vi "GEA2 Send Message.vi"(0 "GEA2 Reference In":refnum<k24>, 1 "Input Data":T1 {"Command" format="%02x"; "Destination" format="%02x"; "Source" format="%02x"}, 2 "Retry Count":u32=3, 11 "Error In":errorcluster) -> (4 "GEA2 Reference Out":refnum<k24>, 15 "Error Out":errorcluster)   [LabVIEW 2016, in "GEA2_Toolkit.lvlib"]
doc: "This VI sends a GEA2 message accross the GEA2 bus."
uses:
  library/GEA2_Toolkit.lvlib
  type defs/Data In.ctl
  C:/Technology Lab/NI-2010/Trunk/Utility/LabVIEW GEA2 Toolkit v1.0.0.0/Appliance.NET/GeaCommunication.dll
  Appliance.NET/GeaCommunication.dll
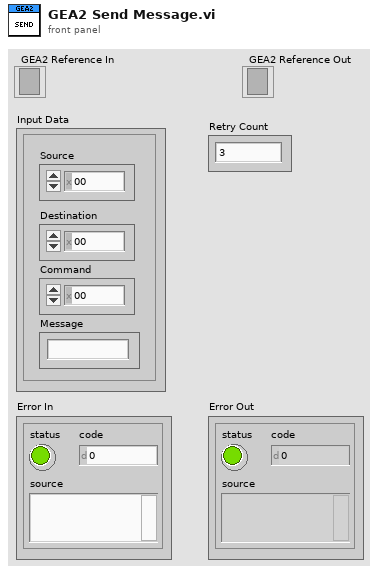
[diagram p1: front panel]
types:
  T1 = typedef "GEA2_Toolkit.lvlib/Data In.ctl" = cluster{"Source":u8, "Destination":u8, "Command":u8, "Message":string}
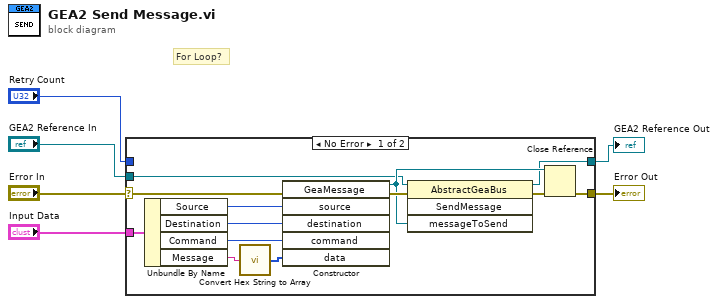
[diagram p0: block diagram]
diagram:
  # "For Loop?"
  n1 = case shown="No Error" "Error In" {
    selector: "Error In" -> [w15 w20]
    tunnel: "GEA2 Reference In" -> [w10 w21]
    tunnel: [w9 w21] -> w1
    tunnel: [w14 w20] -> w6
    tunnel: "Retry Count" -> [_ _]
    tunnel: "Input Data" -> [w19 _]
    frame No Error {
      n2 = Unbundle By Name(w19) -> ("Source"=w18:u8, "Destination"=w17:u8, "Command"=w16:u8, "Message"=w8:string)
      n3 = call "Convert Hex String to Array.vi"("Hex String In"=w8) -> ("Hex Array Out"=w7:u8[])  [unwired: 14 in]
      n4 = constructor class="GeaMessage"(error in=w15, "source"=w18, "destination"=w17, "command"=w16, "data"=w7) -> (reference out=w12:refnum<k24>, error out=w13:errorcluster)  [unwired: 2 in, 5 out]
      n5 = invoke class="AbstractGeaBus" method="SendMessage"(reference=w10, error in=w13, "messageToSend"=w12) -> (reference out=w9:refnum<k24>, error out=w11:errorcluster)  [unwired: 1 in, 2 out]
      n6 = Close Reference(reference=w12, error in (no error)=w11) -> (error out=w14:errorcluster)
    }
    frame Error {
    }
  }
  "Error Out" <- w6
  "GEA2 Reference Out" <- w1
